vi "Write String.vi"(8 "error in (no error)":errorcluster, 10 "String":string, 11 "Log Status in":refnum<class "Log Status.lvclass">) -> (0 "error out":errorcluster, 3 "Log Status out":refnum<class "Log Status.lvclass">)   [LabVIEW 2016, in "Controller Actor.lvlib" / "Log Status.lvclass"]
uses:
  Log Status.lvclass
  Log Status.lvclass/Log Status.ctl
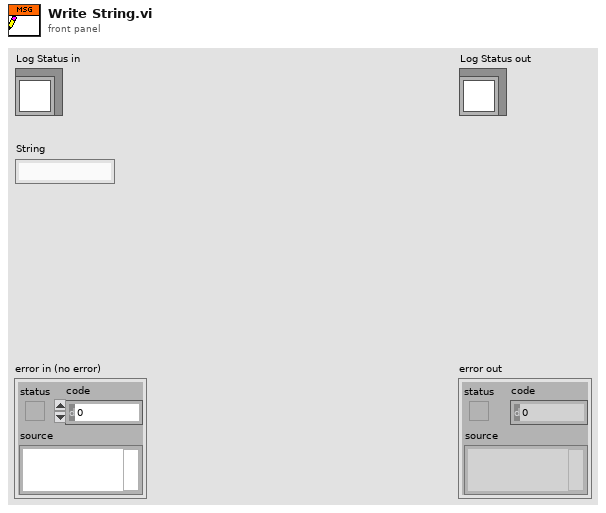
[diagram p1: front panel]
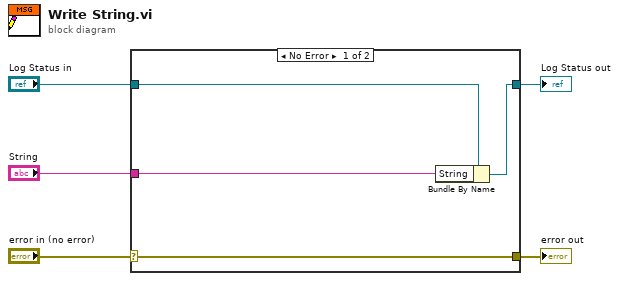
[diagram p0: block diagram]
diagram:
  n1 = case shown="No Error" "error in (no error)" {
    selector: "error in (no error)" -> [w9 w10]
    tunnel: [w9 w10] -> w4
    tunnel: [w7 w11] -> w2
    tunnel: "Log Status in" -> [w8 w11]
    tunnel: "String" -> [w6 _]
    frame No Error {
      n2 = Bundle By Name(cluster=w8, "String"=w6) -> (w7:refnum<class "Log Status.lvclass">)
    }
    frame Error {
    }
  }
  "error out" <- w4
  "Log Status out" <- w2
